vi "Load Bitfile Settings.vi"(8 "error in (no error)":errorcluster, 11 "bitfile path":path) -> (0 "error out":errorcluster, 1 "Bitfile Info":T1, 2 "Valid?":bool, 3 "SLSC version string":string)   [LabVIEW 2014, in "SLSC configuration System Explorer.lvlib"]
uses:
  SLSC configuration System Explorer.lvlib
  Type Defs/SLSC Bitfile Info.ctl
  Shared/Constants.vi
  Shared/SLSC configuration Shared.lvlib
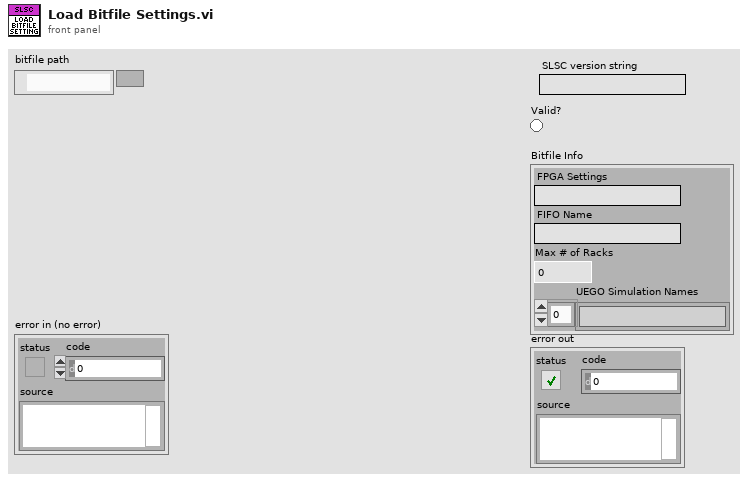
[diagram p1: front panel]
types:
  T1 = typedef "SLSC configuration System Explorer.lvlib/SLSC Bitfile Info.ctl" = cluster{"FPGA Settings":string, "FIFO Name":string, "Max # of Racks":u8, "UEGO Simulation Names":string[]}
  T2 = typedef "SLSC configuration System Explorer.lvlib/SLSC Custom Device Version.ctl" = enum8{"1.0"}
  T3 = typedef "niFpgaBitfileStructure_VI.ctl" = cluster{"Name":string, "RegisterMap":T4[], "Icon":T9}
  T4 = typedef "nirviControlStructure.ctl" = cluster{"Name":string, "Hidden":bool, "Indicator":bool, "Flattened Type":string, "Grouping":cluster{"Grouped":bool, "Member Names":string[], "Member IDs":u32[]}, "Address":u32, "Size":u32, "Class":u32, "Internal":bool, "Typedef":T5, "ID":u32, "Bidirectional":bool, "Synchronous":bool, "Mechanical Action":T6, "Sub Controls":T7[], "Access May Timeout":bool, "Register Node":bool}
  T5 = typedef "nirviTypdefDescription.ctl" = cluster{"Typedef":bool, "Path":path}
  T6 = typedef "nirviMechanicalAction.ctl" = enum8{"Switch When Pressed", "Switch When Released", "Switch Until Released", "Latch When Pressed", "Latch When Released", "Latch Until Released"}
  T7 = typedef "nirviSubControlStructure.ctl" = cluster{"Name":string, "flattened Type":string, "Cluster Information":T8, "Typedef":T5}
  T8 = typedef "nirviClusterElementControl.ctl" = cluster{"Name Hierarchy":string[], "Item Order":u32[]}
  T9 = typedef "imagedata.ctl" = cluster{"image type":i32, "image depth":i32, "image":u8[], "mask":u8[], "colors":u32[], "Rectangle":cluster{"left":i16, "top":i16, "right":i16, "bottom":i16}}
  T10 = typedef "SLSC configuration System Explorer.lvlib/Register Types.ctl" = enum16{"SLSC Settings", "# of Racks", "SPI FIFO Name", "UEGO Calibration"}
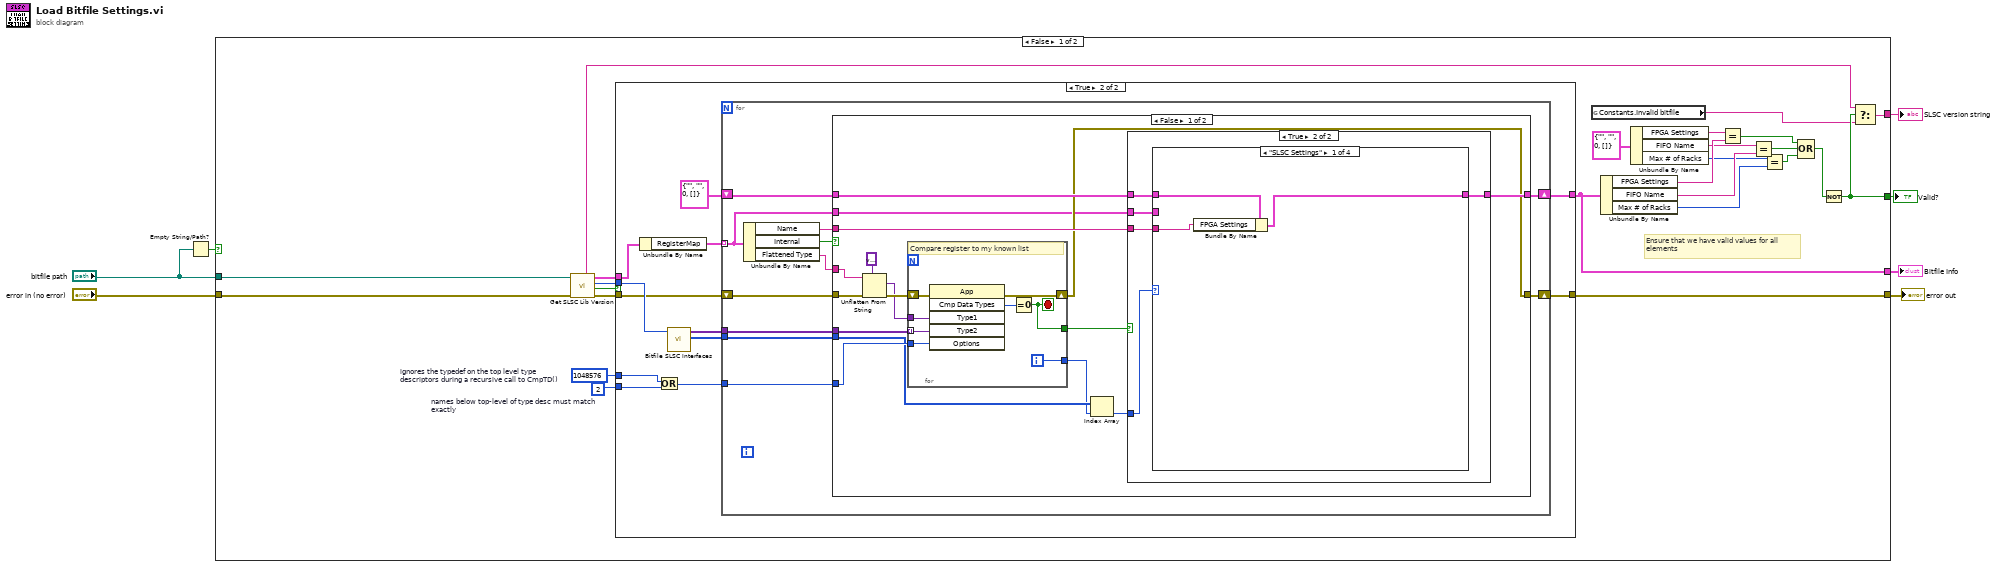
[diagram p0: block diagram]
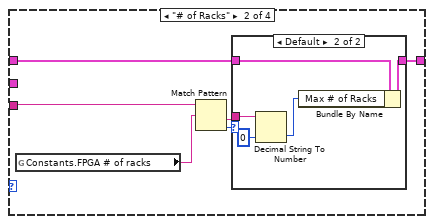
[diagram p4: hidden frame]
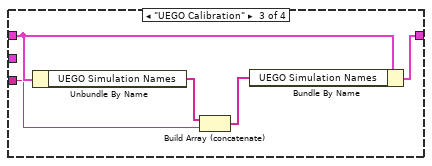
[diagram p6: hidden frame]
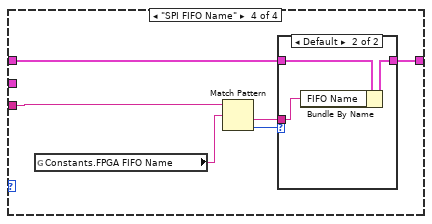
[diagram p7: hidden frame]
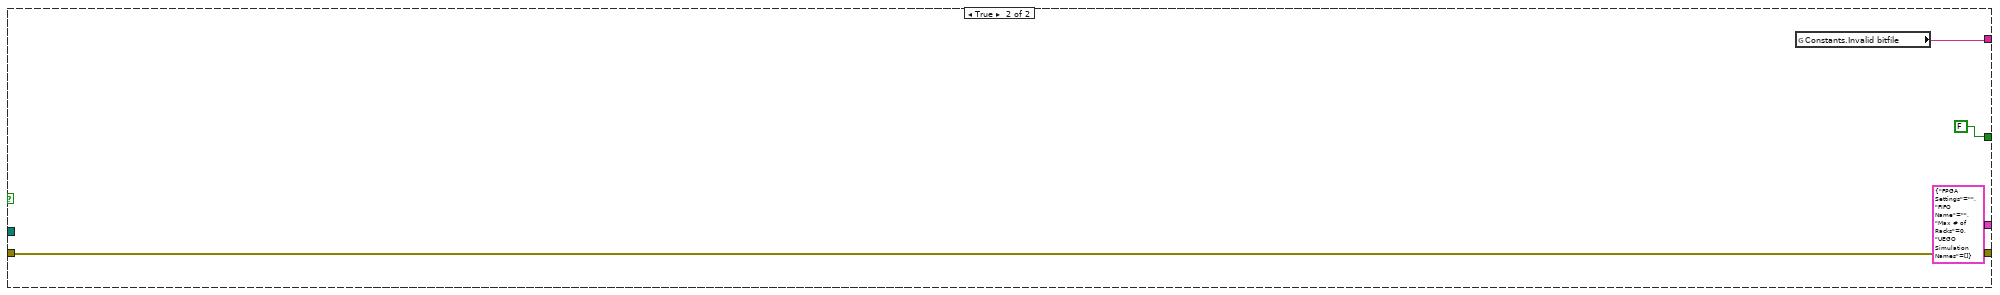
[diagram p10: hidden frame]
diagram:
  n1 = Empty String/Path?(string/path="bitfile path") -> (empty?=w1:bool)
  n2 = case shown="False" w1 {
    tunnel: [w19 T1 {"FPGA Settings"="", "FIFO Name"="", "Max # of Racks"=0, "UEGO Simulation Names"=[]} ("Cluster")] -> w7
    tunnel: "error in (no error)" -> [w27 w122]
    tunnel: [w26 w122] -> w5
    tunnel: [w25 FALSE] -> w4
    tunnel: [w22 w120] -> w3
    tunnel: "bitfile path" -> [w21 _]
    frame False {
      w28 = 2  # names below top-level of type desc must match exactly
      w29 = 1048576  # ignores the typedef on the top level type descriptors during a recursive call to CmpTD()
      # "Ensure that we have valid values for all\nelements"
      n3 = call "Get SLSC Lib Version.vi"("error in (no error)"=w27, "bitfile path"=w21) -> ("error out"=w30:errorcluster, "valid bitfile"=w32:bool, "SLSC version enum"=w31:T2, "vi info"=w8:T3, "SLSC version string"=w23:string)  [unwired: 5 in]
      n4 = case shown="True" w32 {
        tunnel: w31 -> [_ w45]
        tunnel: w8 -> [_ w44]
        tunnel: w30 -> [w33 w40]
        tunnel: w29 -> [_ w39]
        tunnel: w28 -> [_ w38]
        tunnel: [_ w35] -> w19
        tunnel: [w33 w34] -> w26
        frame False {
        }
        frame True {
          n5 = Unbundle By Name(w44) -> ("RegisterMap"=w43:T4[])
          n6 = Or(x=w39, y=w38) -> (x .or. y?=w37:i32)
          n7 = call "Bitfile SLSC Interfaces.vi"("SLSC CD Version"=w45) -> ("IP Types"=w41:T10[], "IP Interface"=w42:variant[])  [unwired: 9 in]
          n8 = for {
            tunnel: w43 -> [w46] mode=indexing
            tunnel: w42 -> [w53]
            tunnel: w41 -> [w52]
            tunnel: w37 -> [w51]
            shift-right: [w48] -> w35
            shift-left: T1 {"FPGA Settings"="", "FIFO Name"="", "Max # of Racks"=0, "UEGO Simulation Names"=[]} ("Cluster") -> [w50]
            shift-right: [w47] -> w34
            shift-left: w40 -> [w54]
            n9 = Unbundle By Name(w46) -> ("Name"=w49:string, "Internal"=w56:bool, "Flattened Type"=w55:string)
            n10 = case shown="False" w56 {
              tunnel: w55 -> [w69 _]
              tunnel: w54 -> [w68 w117]
              tunnel: w53 -> [w67 _]
              tunnel: w52 -> [w65 _]
              tunnel: w51 -> [w66 _]
              tunnel: w50 -> [w61 w118]
              tunnel: w49 -> [w60 _]
              tunnel: [w59 w118] -> w48
              tunnel: [w58 w117] -> w47
              tunnel: w46 -> [w57 _]
              frame False {
                n11 = Unflatten From String(type=variant ("Variant"), binary string=w69, error in (no error)=w68) -> (value=w70:variant, error out=w72:errorcluster)  [unwired: 3 out]
                n12 = for {
                  shift-right: [w115] -> w58
                  shift-left: w72 -> [w116]
                  tunnel: w70 -> [w113]
                  tunnel: w67 -> [w112] mode=indexing
                  tunnel: [w111] -> w63
                  tunnel: [w110] -> w64
                  tunnel: w66 -> [w109]
                  i -> [w110]
                  stop <- w111 stop-if-true
                  # "Compare register to my known list"
                  n13 = invoke class="App" method="Cmp Data Types"(error in=w116, "Type1"=w113, "Type2"=w112, "Options"=w109) -> (error out=w115:errorcluster, "Compare Data Types"=w114:i32)  [unwired: 2 in, 4 out]
                  n14 = Equal To 0?(x=w114) -> (x = 0?=w111:bool)
                }
                n15 = Index Array(array=w65, index=w64) -> (element=w62:T10)
                n16 = case shown="True" w63 {
                  tunnel: w62 -> [_ w78]
                  tunnel: w61 -> [w73 w77]
                  tunnel: w60 -> [_ w76]
                  tunnel: [w73 w75] -> w59
                  tunnel: w57 -> [_ w74]
                  frame False {
                  }
                  frame True {
                    n17 = case shown="\"SLSC Settings\"" w78 {
                      tunnel: w77 -> [w81 w84 w98 w104]
                      tunnel: w76 -> [w80 w83 w95 w102]
                      tunnel: [w79 w85 w97 w103] -> w75
                      tunnel: w74 -> [_ _ _ _]
                      frame "SLSC Settings" {
                        n18 = Bundle By Name(cluster=w81, "FPGA Settings"=w80) -> (w79:T1)
                      }
                      frame "# of Racks" {
                        n19 = global read "Constants.vi" "Constants.FPGA # of racks"() -> (w87:string)
                        n20 = Match Pattern(string=w83, regular expression=w87) -> (after substring=w82:string, offset past match=w86:i32)  [unwired: 1 in, 2 out]
                        n21 = case shown="Default" w86 {
                          tunnel: w84 -> [w88 w93]
                          tunnel: [w88 w92] -> w85
                          tunnel: w82 -> [_ w91]
                          frame -1 {
                          }
                          frame Default {
                            n22 = Decimal String To Number(string=w91, default (0L)=u8 0 ("default (0 I32)")) -> (number=w90:u8)  [unwired: 1 in, 1 out]
                            n23 = Bundle By Name(cluster=w93, "Max # of Racks"=w90) -> (w92:T1)
                          }
                        }
                      }
                      frame "UEGO Calibration" {
                        n24 = Unbundle By Name(w98) -> ("UEGO Simulation Names"=w96:string[])
                        n25 = Build Array (concatenate)(w96, w95) -> (w94:string[])
                        n26 = Bundle By Name(cluster=w98, "UEGO Simulation Names"=w94) -> (w97:T1)
                      }
                      frame "SPI FIFO Name" {
                        n27 = global read "Constants.vi" "Constants.FPGA FIFO Name"() -> (w100:string)
                        n28 = Match Pattern(string=w102, regular expression=w100) -> (after substring=w101:string, offset past match=w99:i32)  [unwired: 1 in, 2 out]
                        n29 = case shown="Default" w99 {
                          tunnel: w104 -> [w105 w108]
                          tunnel: [w105 w107] -> w103
                          tunnel: w101 -> [_ w106]
                          frame -1 {
                          }
                          frame Default {
                            n30 = Bundle By Name(cluster=w108, "FIFO Name"=w106) -> (w107:T1)
                          }
                        }
                      }
                    }
                  }
                }
              }
              frame True {
              }
            }
          }
        }
      }
      n31 = global read "Constants.vi" "Constants.Invalid bitfile"() -> (w24:string)
      n32 = Unbundle By Name(w19) -> ("FPGA Settings"=w17:string, "FIFO Name"=w15:string, "Max # of Racks"=w13:u8)
      n33 = Unbundle By Name(T1 {"FPGA Settings"="", "FIFO Name"="", "Max # of Racks"=0, "UEGO Simulation Names"=[]} ("Cluster")) -> ("FPGA Settings"=w18:string, "FIFO Name"=w16:string, "Max # of Racks"=w14:u8)
      n34 = Equal?(x=w18, y=w17) -> (x = y?=w12:bool)
      n35 = Equal?(x=w16, y=w15) -> (x = y?=w11:bool)
      n36 = Equal?(x=w14, y=w13) -> (x = y?=w10:bool)
      n37 = Compound Arithmetic op=OR(w12, w11, w10) -> (w9:bool)
      n38 = Not(x=w9) -> (.not. x?=w25:bool)
      n39 = Select(t=w23, s=w25, f=w24) -> (s? t:f=w22:string)
    }
    frame True {
      n40 = global read "Constants.vi" "Constants.Invalid bitfile"() -> (w120:string)
    }
  }
  "SLSC version string" <- w3
  "Bitfile Info" <- w7
  "Valid?" <- w4
  "error out" <- w5
